vi "Step mm con.vi"(8 "error in (no error)":errorcluster, 9 "mm in":dbl, 10 "Step in":i32, 11 "Lifter_motor in":refnum<class "Lifter_motor.lvclass">) -> (0 "error out":errorcluster, 1 "step out":i32, 2 "mm out":dbl, 3 "Lifter_motor out":refnum<class "Lifter_motor.lvclass">)   [LabVIEW 2019, in "Lifter_motor.lvclass"]
uses:
  Lifter_motor.lvclass
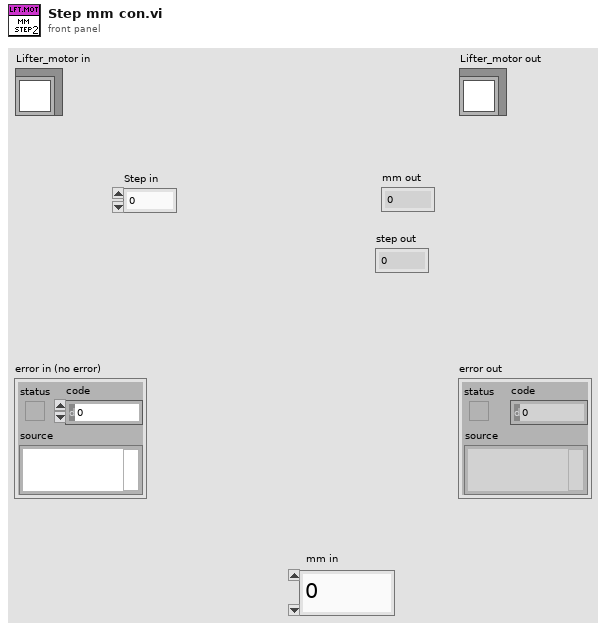
[diagram p1: front panel]
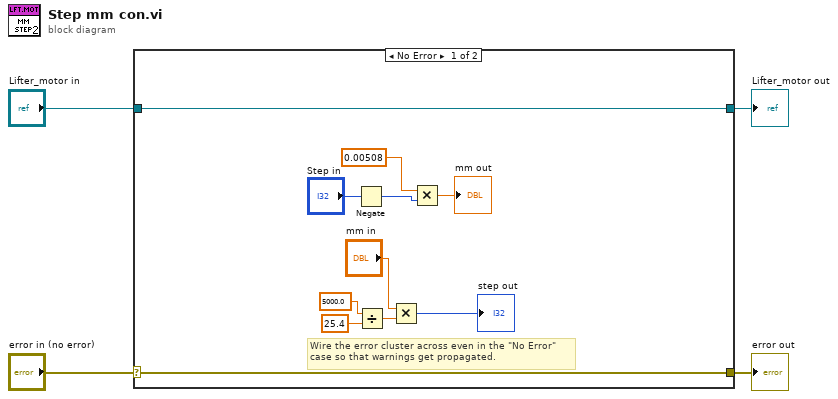
[diagram p0: block diagram]
diagram:
  n1 = case shown="No Error" "error in (no error)" {
    selector: "error in (no error)" -> [w14 w17]
    tunnel: [w14 w17] -> w3
    tunnel: [w15 w16] -> w1
    tunnel: "Lifter_motor in" -> [w15 w16]
    frame No Error {
      # "Wire the error cluster across even in the \"No Error\"\ncase so that warnings get propagated."
      n2 = Negate(x="Step in") -> (-x=w13:i32)
      n3 = Divide(x=5000.0, y=25.4) -> (x/y=w9:dbl)
      n4 = Multiply(x="mm in", y=w9) -> (x*y=→"step out":i32)
      n5 = Multiply(x=0.00508, y=w13) -> (x*y=→"mm out":dbl)
    }
    frame Error {
    }
  }
  "error out" <- w3
  "Lifter_motor out" <- w1
